vi "Facade.vi"(0 "Data In":T4, 2 "Display State In":T2, 3 "Container State":T3) -> (6 "Data Out":T4, 7 "Display State Out":T2, 8 "Action":T1)   [LabVIEW 2020, in "MixerSlider.xctl"]
uses:
  MixerSlider.xctl
  Data.ctl
  <vilib>/_xctls/Container State.ctl
  State.ctl
  <vilib>/_xctls/Action.ctl
  <vilib>/_xctls/XControlSupport.lvlib
panel:
  in  "Mute":bool
  in  "Slider":dbl(slide)
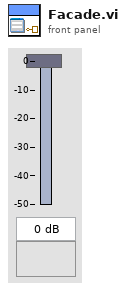
[diagram p1: front panel]
types:
  T1 = typedef "XControlSupport.lvlib/Action.ctl" = cluster{"Data Changed?":bool, "State Changed?":bool, "Action Name":string}
  T2 = typedef "MixerSlider.xctl/State.ctl" = cluster{"url":string, "muted":bool, "slider enabled":bool, "mute enabled":bool, "action":string}
  T3 = typedef "XControlSupport.lvlib/Container State.ctl" = cluster{"Indicator?":bool, "Run Mode?":bool, " Refnum":refnum<vi>}
  T4 = typedef "MixerSlider.xctl/Data.ctl" = dbl
  T5 = enum8{"Enabled", "Disabled", "Disabled and Grayed Out"}
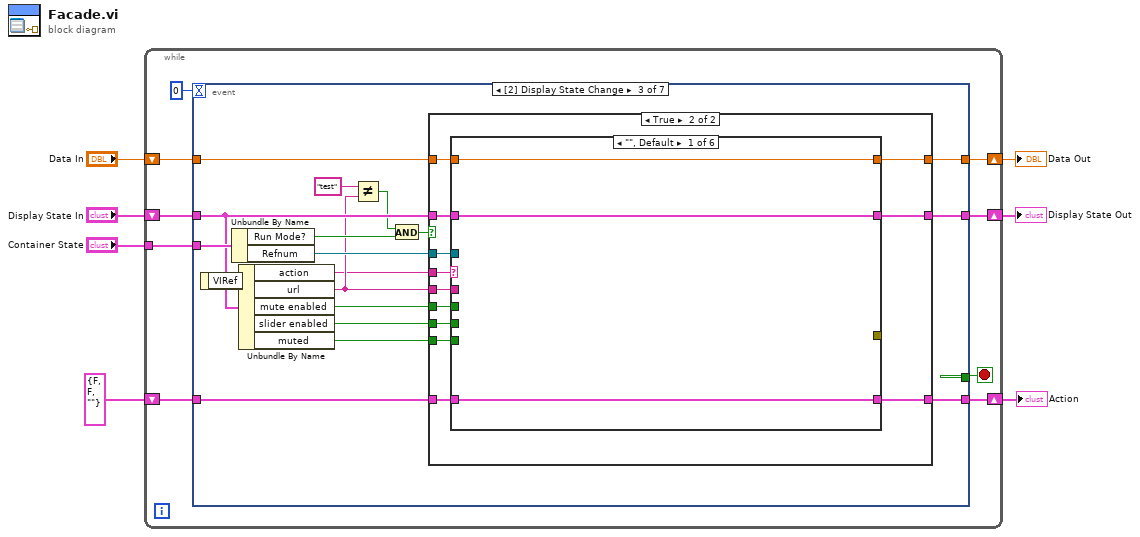
[diagram p0: block diagram]
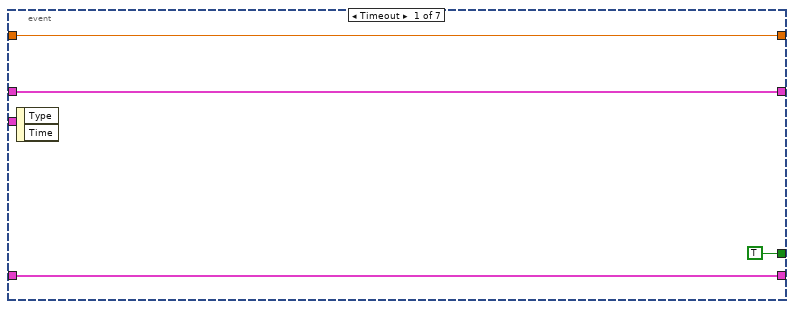
[diagram p2: hidden frame]
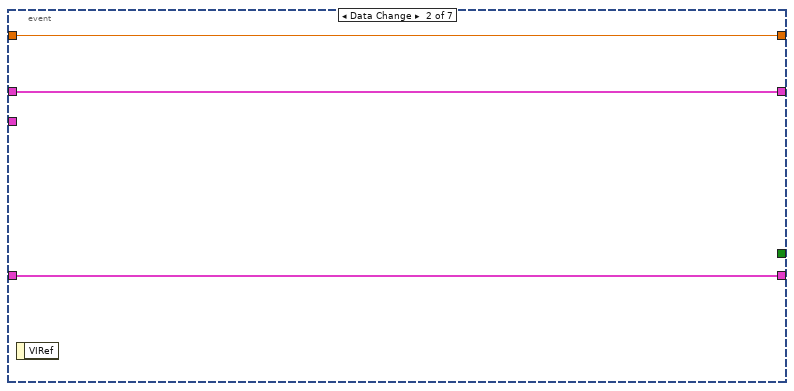
[diagram p3: hidden frame]
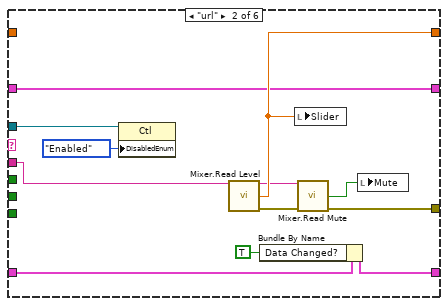
[diagram p5: hidden frame]
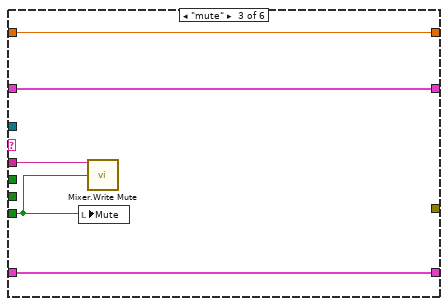
[diagram p6: hidden frame]
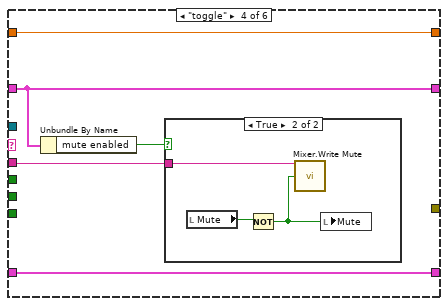
[diagram p7: hidden frame]
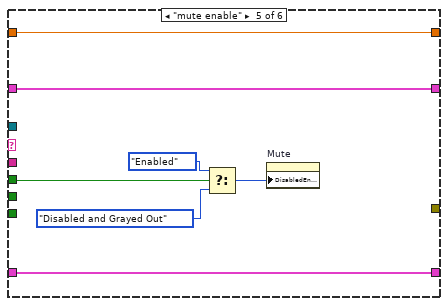
[diagram p9: hidden frame]
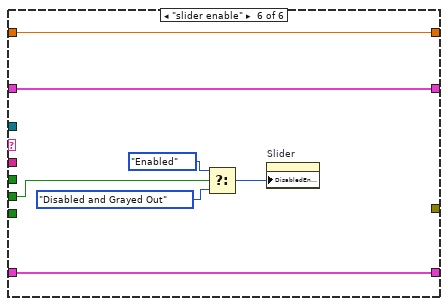
[diagram p10: hidden frame]
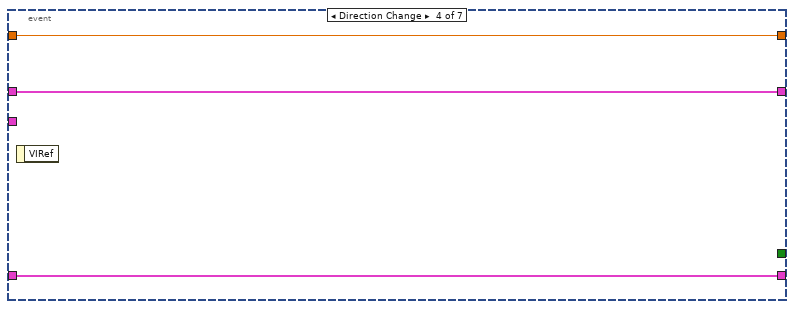
[diagram p11: hidden frame]
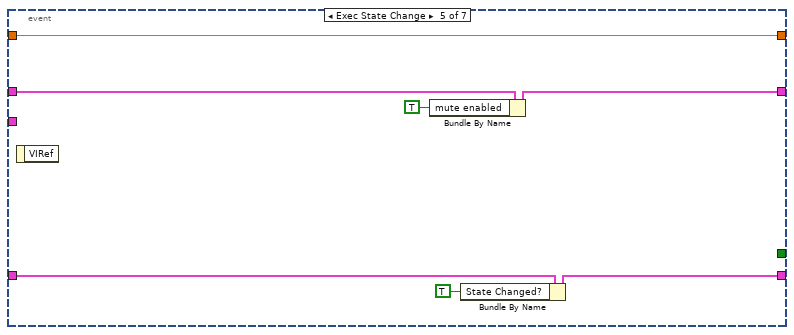
[diagram p12: hidden frame]
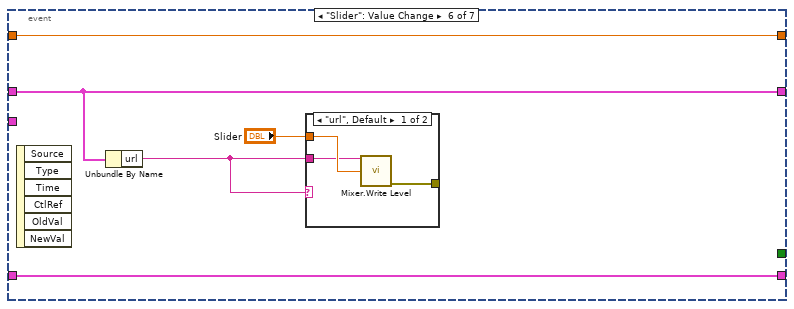
[diagram p13: hidden frame]
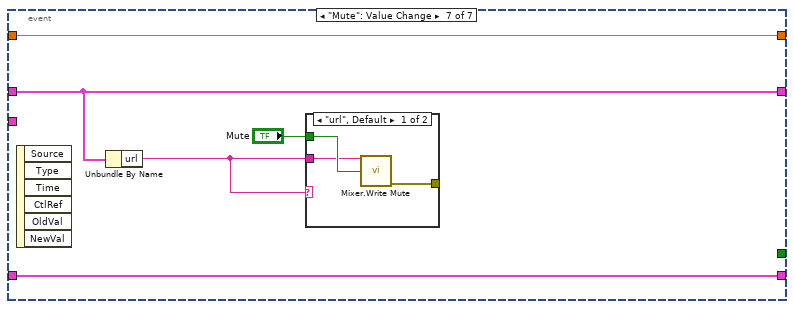
[diagram p15: hidden frame]
diagram:
  n1 = while {
    shift-right: [w15] -> w4
    shift-left: "Display State In" -> [w16]
    tunnel: "Container State" -> [w12]
    shift-right: [w10] -> w7
    shift-left: "Data In" -> [w11]
    shift-right: [w8] -> w2
    shift-left: T1 {"Data Changed?"=FALSE, "State Changed?"=FALSE, "Action Name"=""} ("Action") -> [w9]
    stop <- w14 stop-if-true
    n2 = event shown="[2] Display State Change" {
      selector: _ -> [_ _ _ _ _ _ _]
      dyn-events: _ -> [_ _ _ _ _ _ _]
      timeout: 0 -> [_ _ _ _ _ _ _]
      tunnel: w16 -> [w18 w22 w33 w100 w107 w110 w118]
      tunnel: [w18 w22 w30 w100 w104 w110 w118] -> w15
      tunnel: [TRUE _ _ _ _ _ _] -> w14
      tunnel: w12 -> [_ _ w37 _ _ _ _]
      tunnel: w11 -> [w17 w23 w32 w99 w106 w112 w120]
      tunnel: [w17 w23 w31 w99 w106 w112 w120] -> w10
      tunnel: [w19 w21 w34 w98 w102 w111 w119] -> w8
      tunnel: w9 -> [w19 w21 w35 w98 w105 w111 w119]
      event Timeout {
        n3 = event-data() -> ()  [unwired: 1 in, 2 out]
      }
      event Data Change {
        n4 = event-data() -> ()  [unwired: 1 in, 1 out]
      }
      event Display State Change {
        n5 = event-data() -> ()  [unwired: 1 in, 1 out]
        n6 = Unbundle By Name(w37) -> ("Run Mode?"=w29:bool, "Refnum"=w36:refnum<vi>)
        n7 = Unbundle By Name(w33) -> ("action"=w24:string, "url"=w28:string, "mute enabled"=w40:bool, "slider enabled"=w39:bool, "muted"=w38:bool)
        n8 = Not Equal?(x="test", y=w28) -> (x != y?=w25:bool)
        n9 = And(x=w25, y=w29) -> (x .and. y?=w26:bool)
        n10 = case shown="True" w26 {
          tunnel: w28 -> [_ w55]
          tunnel: w40 -> [_ w54]
          tunnel: w39 -> [_ w53]
          tunnel: w38 -> [_ w52]
          tunnel: w24 -> [_ w51]
          tunnel: w36 -> [_ w50]
          tunnel: w35 -> [w41 w49]
          tunnel: [w41 w48] -> w34
          tunnel: w33 -> [w42 w47]
          tunnel: w32 -> [w43 w46]
          tunnel: [w43 w45] -> w31
          tunnel: [w42 w44] -> w30
          frame False {
          }
          frame True {
            n11 = case shown="\"\", Default" w51 {
              tunnel: w54 -> [_ _ _ _ w84 _]
              tunnel: w53 -> [_ _ _ _ _ w91]
              tunnel: w52 -> [_ _ w71 _ _ _]
              tunnel: w55 -> [_ w63 w72 w78 _ _]
              tunnel: w50 -> [_ w70 _ _ _ _]
              tunnel: w49 -> [w58 w68 w75 w80 w87 w94]
              tunnel: [w58 w67 w75 w80 w87 w94] -> w48
              tunnel: w47 -> [w56 w64 w73 w77 w85 w92]
              tunnel: w46 -> [w57 _ w74 w79 w86 w93]
              tunnel: [w57 w65 w74 w79 w86 w93] -> w45
              tunnel: [w56 w64 w73 w77 w85 w92] -> w44
              tunnel: [_ w61 _ _ _ _] -> _
              frame "", Default {
              }
              frame "url" {
                n12 = property class="Ctl"(reference=w70, "DisabledEnum"=T5."Enabled" ("Disabled")) -> ()  [unwired: 1 in, 2 out]
                n13 = call "Mixer.Read Level.vi"("baseURL"=w63) -> ("baseURL out"=w60:string, "value"=w65:dbl, "error out"=w62:errorcluster)  [unwired: 12 in]
                n14 = Bundle By Name(cluster=w68, "Data Changed?"=TRUE) -> (w67:T1)
                n15 = local write "Slider"(w65) -> ()
                n16 = call "Mixer.Read Mute.vi"("baseURL"=w60, "error in (no error)"=w62) -> ("value"=w59:bool, "error out"=w61:errorcluster)  [unwired: 11 in, 1 out]
                n17 = local write "Mute"(w59) -> ()
              }
              frame "mute" {
                n18 = local write "Mute"(w71) -> ()
                n19 = call "Mixer.Write Mute.vi"("baseURL"=w72, "mute"=w71) -> ()  [unwired: 13 in, 1 out]
              }
              frame "toggle" {
                n20 = Unbundle By Name(w77) -> ("mute enabled"=w76:bool)
                n21 = case shown="True" w76 {
                  tunnel: w78 -> [_ w83]
                  frame False {
                  }
                  frame True {
                    n22 = local read "Mute"() -> (w82:bool)
                    n23 = Not(x=w82) -> (.not. x?=w81:bool)
                    n24 = call "Mixer.Write Mute.vi"("baseURL"=w83, "mute"=w81) -> ()  [unwired: 13 in, 1 out]
                    n25 = local write "Mute"(w81) -> ()
                  }
                }
              }
              frame "mute enable" {
                n26 = Select(t=T5."Enabled" ("Disabled"), s=w84, f=T5."Disabled and Grayed Out" ("Disabled")) -> (s? t:f=w89:T5)
                n27 = property on="Mute" class="Bool (strict)"("DisabledEnum"=w89) -> ()  [unwired: 2 in, 2 out]
              }
              frame "slider enable" {
                n28 = Select(t=T5."Enabled" ("Disabled"), s=w91, f=T5."Disabled and Grayed Out" ("Disabled")) -> (s? t:f=w96:T5)
                n29 = property on="Slider" class="Slide (strict)"("DisabledEnum"=w96) -> ()  [unwired: 2 in, 2 out]
              }
            }
          }
        }
      }
      event Direction Change {
        n30 = event-data() -> ()  [unwired: 1 in, 1 out]
      }
      event Exec State Change {
        n31 = event-data() -> ()  [unwired: 1 in, 1 out]
        n32 = Bundle By Name(cluster=w107, "mute enabled"=TRUE) -> (w104:T2)
        n33 = Bundle By Name(cluster=w105, "State Changed?"=TRUE) -> (w102:T1)
      }
      event "Slider": Value Change {
        n34 = event-data() -> ()  [unwired: 1 in, 6 out]
        n35 = Unbundle By Name(w110) -> ("url"=w108:string)
        n36 = case shown="\"url\", Default" w108 {
          tunnel: w108 -> [w114 _]
          tunnel: "Slider" -> [w115 _]
          tunnel: [w113 _] -> _
          frame "url", Default {
            n37 = call "Mixer.Write Level.vi"("baseURL"=w114, "value"=w115) -> ("error out"=w113:errorcluster)  [unwired: 12 in, 1 out]
          }
          frame "test" {
          }
        }
      }
      event "Mute": Value Change {
        n38 = event-data() -> ()  [unwired: 1 in, 6 out]
        n39 = Unbundle By Name(w118) -> ("url"=w116:string)
        n40 = case shown="\"url\", Default" w116 {
          tunnel: w116 -> [w122 _]
          tunnel: "Mute" -> [w123 _]
          tunnel: [w121 _] -> _
          frame "url", Default {
            n41 = call "Mixer.Write Mute.vi"("baseURL"=w122, "mute"=w123) -> ("error out"=w121:errorcluster)  [unwired: 13 in]
          }
          frame "test" {
          }
        }
      }
    }
  }
  "Display State Out" <- w4
  "Data Out" <- w7
  "Action" <- w2
